vi "AWS-S3-BeginDownload.vi"(0 "AWS-S3-API":refnum<class "AWS-S3-API.lvclass">, 5 "Object Key":string, 7 "Object Bucket":string, 9 "Destination Path (Local)":path, 11 "error in":errorcluster, 12 "Object VersionID":string) -> (4 "AWS-S3-API out":refnum<class "AWS-S3-API.lvclass">, 15 "error out":errorcluster)   [LabVIEW 2012, in "AWS-S3-API.lvclass"]
uses:
  AWS-S3-API.lvclass
  AWS-S3-Transfer-Progress.ctl
  AWS-S3-Transfer-Header.ctl
  AWS-S3-API.lvclass/AWS-S3-API.ctl
  C:/Users/Jack/repo/visualize/Dependencies/aws/AWS-SDK/AWSSDK.dll
  AWS-SDK/AWSSDK.dll
panel:
  # "Inputs"
  # "Outputs"
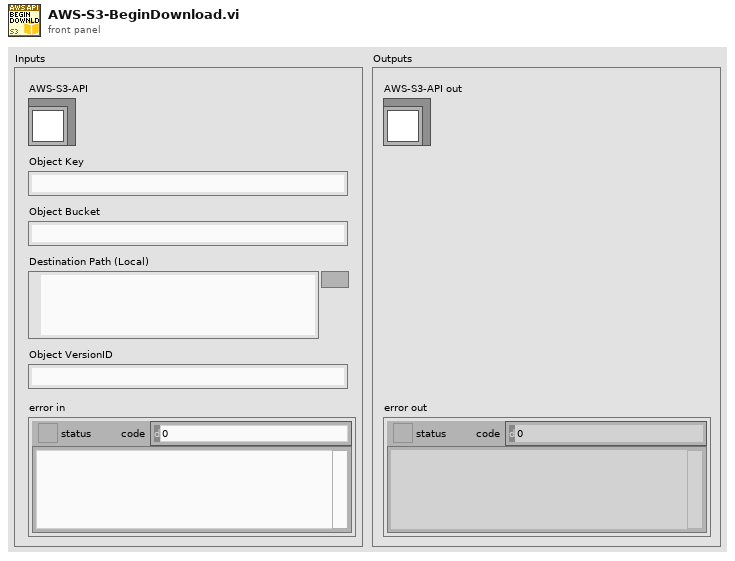
[diagram p1: front panel]
types:
  T1 = cluster{"Initial Timestamp":u32, "Transfer Progress":refnum<user-event>, "Destination Path (Local)":path}
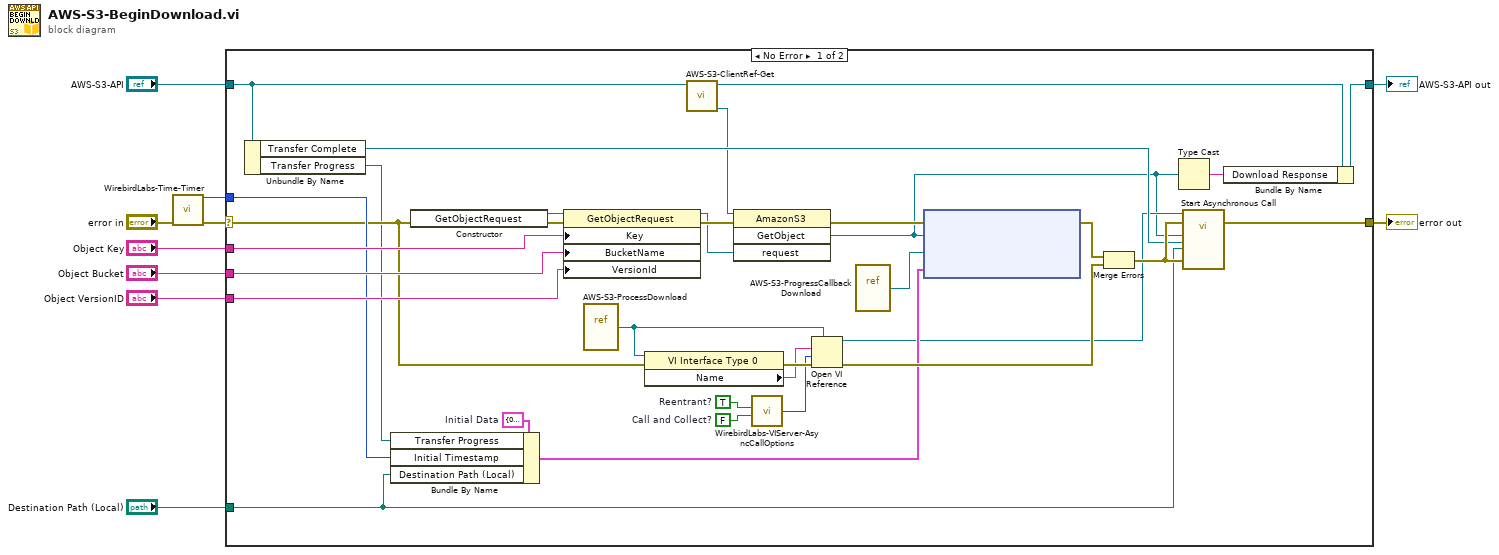
[diagram p0: block diagram]
diagram:
  n1 = call "WirebirdLabs-Time-Timer.vi"("error in"="error in") -> ("Timer (msec)"=w3:u32, "error out"=w1:errorcluster)  [unwired: 10 in, 3 out]
  n2 = case shown="No Error" w1 {
    selector: w1 -> [w25 w45]
    tunnel: [w16 w45] -> w10
    tunnel: [w17 w44] -> w8
    tunnel: "AWS-S3-API" -> [w14 w44]
    tunnel: "Destination Path (Local)" -> [w24 _]
    tunnel: "Object Key" -> [w38 _]
    tunnel: "Object Bucket" -> [w37 _]
    tunnel: "Object VersionID" -> [w36 _]
    tunnel: w3 -> [w27 _]
    frame No Error {
      w19 = FALSE  # Call and Collect?
      w20 = TRUE  # Reentrant?
      w31 = T1 {"Initial Timestamp"=0, "Transfer Progress"=refnum, "Destination Path (Local)"=path ""}  # Initial Data
      n3 = Unbundle By Name(w14) -> ("Transfer Complete"=w32:refnum<user-event>, "Transfer Progress"=w21:refnum<user-event>)
      n4 = Bundle By Name(cluster=w31, "Transfer Progress"=w21, "Initial Timestamp"=w27, "Destination Path (Local)"=w24) -> (w30:T1)
      n5 = constructor class="GetObjectRequest"(error in=w25) -> (reference out=w39:refnum<k24>, error out=w42:errorcluster)  [unwired: 2 in, 1 out]
      n6 = property class="GetObjectRequest"(reference=w39, error in=w42, "Key"=w38, "BucketName"=w37, "VersionId"=w36) -> (reference out=w23:refnum<k24>, error out=w41:errorcluster)
      n7 = vi-ref "AWS-S3-ProcessDownload.vi"() -> (w33:refnum<vi>)
      n8 = property class="VI Interface Type 0"(reference=w33, error in=w25) -> (error out=w35:errorcluster, "Name"=w34:string)  [unwired: 1 out]
      n9 = call "AWS-S3-ClientRef-Get.vi"("AWS-S3-API"=w14) -> ("S3 Client ref"=w15:refnum<k24>, "AWS-S3-API out"=w13:refnum<class "AWS-S3-API.lvclass">)  [unwired: 9 in]
      n10 = invoke class="AmazonS3" method="GetObject"(reference=w15, error in=w41, "request"=w23) -> (error out=w26:errorcluster, "GetObject"=w12:refnum<k24>)  [unwired: 1 in, 2 out]
      n11 = call "WirebirdLabs-VIServer-AsyncCallOptions.vi"("Call and Collect?"=w19, "Reentrant?"=w20) -> ("Open VI Ref Options"=w18:i32)  [unwired: 4 in]
      n12 = Open VI Reference(type specifier VI Refnum (for type only)=w33, vi path=w34, options=w18, error in (no error)=w35) -> (vi reference=w22:refnum<vi>, error out=w40:errorcluster)  [unwired: 2 in]
      n13 = vi-ref "AWS-S3-ProgressCallbackDownload.vi"() -> ("vi reference"=w29:refnum<vi>)
      n14 = node(w26, w12, w29, w30) -> (w28:errorcluster)  [unwired: 1 in, 1 out]
      n15 = Merge Errors(w28, w40) -> (w43:errorcluster)
      n16 = Type Cast(x=w12) -> (*(type *) &x=w11:string)  [unwired: 1 in]
      n17 = call-by-ref "Start Asynchronous Call"(reference=w22, error in=w43, "Get Object Response"=w12, "Download Complete Event"=w32, "Destination Path (Local)"=w24, "error in"=w43) -> (error out=w16:errorcluster)  [unwired: 12 in, 1 out]
      n18 = Bundle By Name(cluster=w13, "Download Response"=w11) -> (w17:refnum<class "AWS-S3-API.lvclass">)
    }
    frame Error {
    }
  }
  "error out" <- w10
  "AWS-S3-API out" <- w8
